vi "Switch tables test.vi"() -> ()   [LabVIEW 2016]
uses:
  LV-Data/src/LV-Data.PG/LV-Data.PGSQL.lvclass
  <vilib>/addons/_JKI Toolkits/Caraya/classes/Test/Test.lvclass
  <vilib>/addons/_JKI Toolkits/Caraya/classes/Assert/Assert.lvclass
  <vilib>/addons/_JKI Toolkits/Caraya/classes/Assert/Assert Not Error.vi
panel:
  in  "error in (no error) 2":errorcluster
  out "error in (no error)":errorcluster
  out "Data.PG out":refnum<class "LV-Data.PGSQL.lvclass">
  in  "LV-Data.PGSQL in":refnum<class "LV-Data.PGSQL.lvclass">
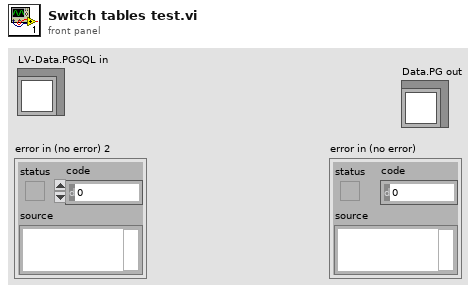
[diagram p1: front panel]
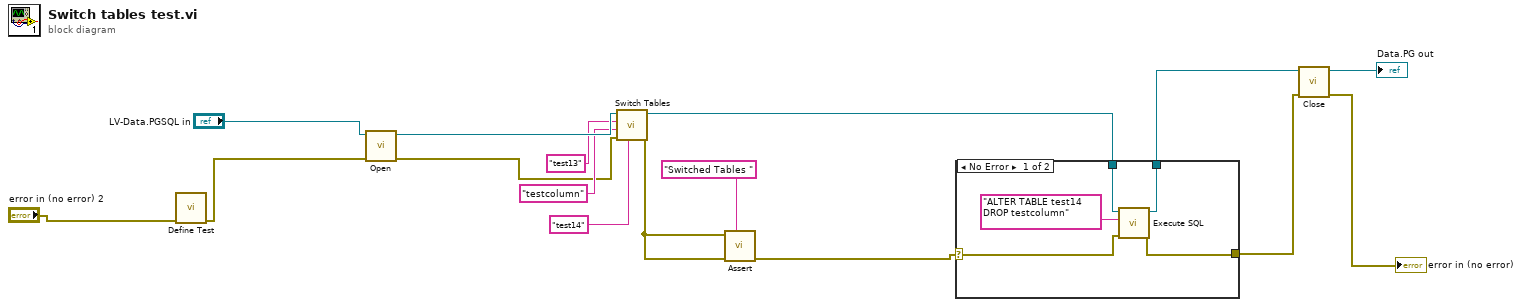
[diagram p0: block diagram]
diagram:
  n1 = call <vilib>:"Define Test.vi"("error in (no error)"="error in (no error) 2") -> ("error out"=w9:errorcluster)  [unwired: 10 in]
  n2 = call-dynamic "Open.vi"("error in (no error)"=w9, "Data.PG in"="LV-Data.PGSQL in") -> ("error out"=w11:errorcluster, "Data.PG out"=w16:refnum<class "LV-Data.PGSQL.lvclass">)  [unwired: 8 in]
  n3 = call "Switch Tables.vi"("New Table"="test14", "error in (no error)"=w11, "Old Column"="testcolumn", "Old Table"="test13", "Data.PG"=w16) -> ("error out"=w8:errorcluster, "Data.PG out"=w4:refnum<class "LV-Data.PGSQL.lvclass">)  [unwired: 4 in, 1 out]
  n4 = call-poly <vilib>:"Assert.vi"("Label"="Switched Tables ", "error in (no error)"=w8, "Not Error?"=w8) -> ("error out"=w3:errorcluster)  [unwired: 8 in]
  n5 = case shown="No Error" w3 {
    selector: w3 -> [w20 w23]
    tunnel: [w19 w23] -> w1
    tunnel: [w21 w22] -> w5
    tunnel: w4 -> [w17 w22]
    frame No Error {
      n6 = call "Execute SQL.vi"("error in"=w20, "SQL"="ALTER TABLE test14 DROP testcolumn", "Data.PG"=w17) -> ("error out"=w19:errorcluster, "Data.PG out"=w21:refnum<class "LV-Data.PGSQL.lvclass">)  [unwired: 6 in, 1 out]
    }
    frame Error {
    }
  }
  n7 = call-dynamic "Close.vi"("error in (no error)"=w1, "Data.PG in"=w5) -> ("error out"=→"error in (no error)":errorcluster, "Data.PG out"=→"Data.PG out":refnum<class "LV-Data.PGSQL.lvclass">)  [unwired: 8 in]
